vi "Temprature warnings.vi"() -> ()   [LabVIEW 2013]
panel:
  out "Warning text":string
  out "Warning?":bool
  in  "Min Temprature":dbl
  in  "Max Temptature":dbl
  in  "Current Temprature":dbl
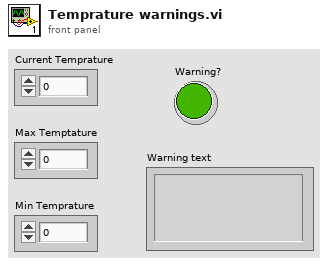
[diagram p1: front panel]
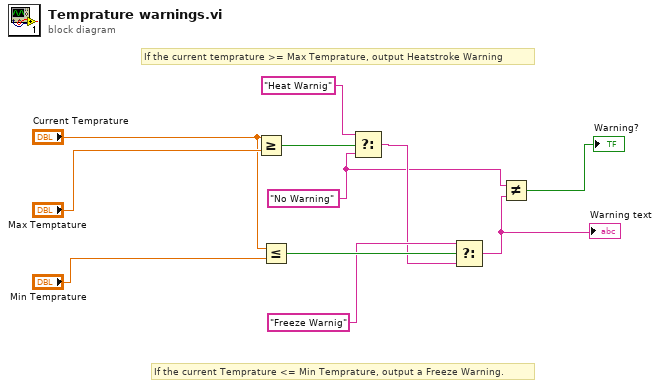
[diagram p0: block diagram]
diagram:
  w1 = "No Warning"
  # "If the current Temprature <= Min Temprature, output a Freeze Warning."
  # "If the current temprature >= Max Temprature, output Heatstroke Warning"
  n1 = Greater Or Equal?(x="Current Temprature", y="Max Temptature") -> (x >= y?=w8:bool)
  n2 = Less Or Equal?(x="Current Temprature", y="Min Temprature") -> (x <= y?=w6:bool)
  n3 = Select(t="Heat Warnig", s=w8, f=w1) -> (s? t:f=w4:string)
  n4 = Select(t="Freeze Warnig", s=w6, f=w4) -> (s? t:f=w2:string)
  "Warning text" <- w2
  n5 = Not Equal?(x=w1, y=w2) -> (x != y?=→"Warning?":bool)
